vi "XIPIN_Accumulator_12_0.vi"   [LabVIEW 2017]
doc: "The Xilinx LogiCORE Accumulator can generate adder- subtractor- and adder/subtractor-based accumulators operating on signed or unsigned input. Inputs range from 1 to 256 bits wide, and outputs, from 1 to 258 bits.\n------------------------------------\n<b>Need License</b> : No"
uses:
  <vilib>/rvi/XilinxIP/XIPIN_XNode/niFpgaXIPIN.xnode
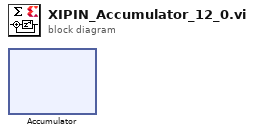
[diagram p0: block diagram]
diagram:
  n1 = xnode ("Accumulator")() -> ()
